vi "Machos.vi"() -> ()   [LabVIEW 2013]
doc: "This example performs a serial port write and a serial port read. The parameters set for the serial port must match the parameters of the connected instrument or device. The VISA Configure Serial Port VI sets the configuration parameters. The front panel displays the controls used to configure the basic parameters, such as baud rate, data bits, and parity. The VI passes the VISA resource name to other VIs that perform operations on that VISA resource. The VISA Write function sends a command to the serial device and the VISA Read function returns data based on the command. The VISA Close function then closes the reference to the serial device. It is important to close the reference; otherwise, further communication through that port might not be possible."
uses:
  <vilib>/Platform/TimedLoop/XDataNode/timing_clust.ctl
  <vilib>/Platform/TimedLoop/XDataNode/nitl_modes.ctl
  <vilib>/Platform/TimedLoop/XDataNode/wakeup.ctl
  <vilib>/Instr/_visa.llb/VISA Configure Serial Port (Instr).vi
  <vilib>/Utility/file.llb/Read From Spreadsheet File (string).vi
  <vilib>/platform/TimedLoop/XDataNode/XDataNode.xnode
  <vilib>/Platform/TimedLoop/XDataNode/XDNodeRunTimeDep.lvlib
panel:
  out "Total":string[](array[string])
  in  "Abrir arnés":bool
  out "Etiquetas":string[](array[string])
  out "Entradas":u8[](array[numeric])
  out "Total":bool[](array[boolean])
  out "Test?":bool[](array[boolean])
  in  "OUTPUT Pin":u8=1 min=1 max=32 step=1
  in  "Puerto":refnum<visa-resource-name>
  out "OK?":bool
  in  "stop":bool
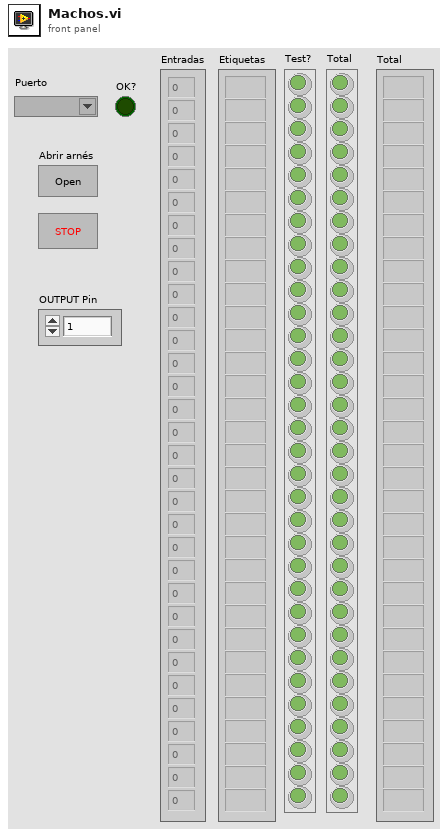
[diagram p1: front panel]
types:
  T1 = typedef "XDNodeRunTimeDep.lvlib/timing_clust.ctl" = cluster{"Expected End [f-1]":u64, "Actual End [f-1]":u64, "Finished Late? [f-1]":bool, "Expected End [i-1]":u64, "Actual End [i-1]":u64, "Finished Late? [i-1]":bool, "Expected Start [i]":u64, "Actual Start [i]":u64, "Expected Start [f]":u64, "Actual Start [f]":u64, "Source Name":string, "Structure Name":string, "Period":i64, "Deadline":i64, "Offset":i64, "Start":i64, "Priority":i32, "Timeout":i32, "Mode":T2, "Wakeup Reason":T3, "Error":errorcluster, "Source Type":string, "Secondary Source Type":string, "Global End Time":u64, "Global Start Time":u64, "Frame Duration":u64, "Iteration Duration":u64, "Assigned CPU":i32, "I/O Scan Engine Mode":u32}
  T2 = typedef "XDNodeRunTimeDep.lvlib/nitl_modes.ctl" = enum32{"No Change", "Process missed periods, maintain original phase", "Discard missed periods, maintain original phase", "Process missed periods, ignore original phase", "Discard missed periods, ignore original phase"}
  T3 = typedef "XDNodeRunTimeDep.lvlib/wakeup.ctl" = enum32{"Normal", "Aborted", "Asynchronous wakeup", "Timing source error", "Timed loop error", "Timeout"}
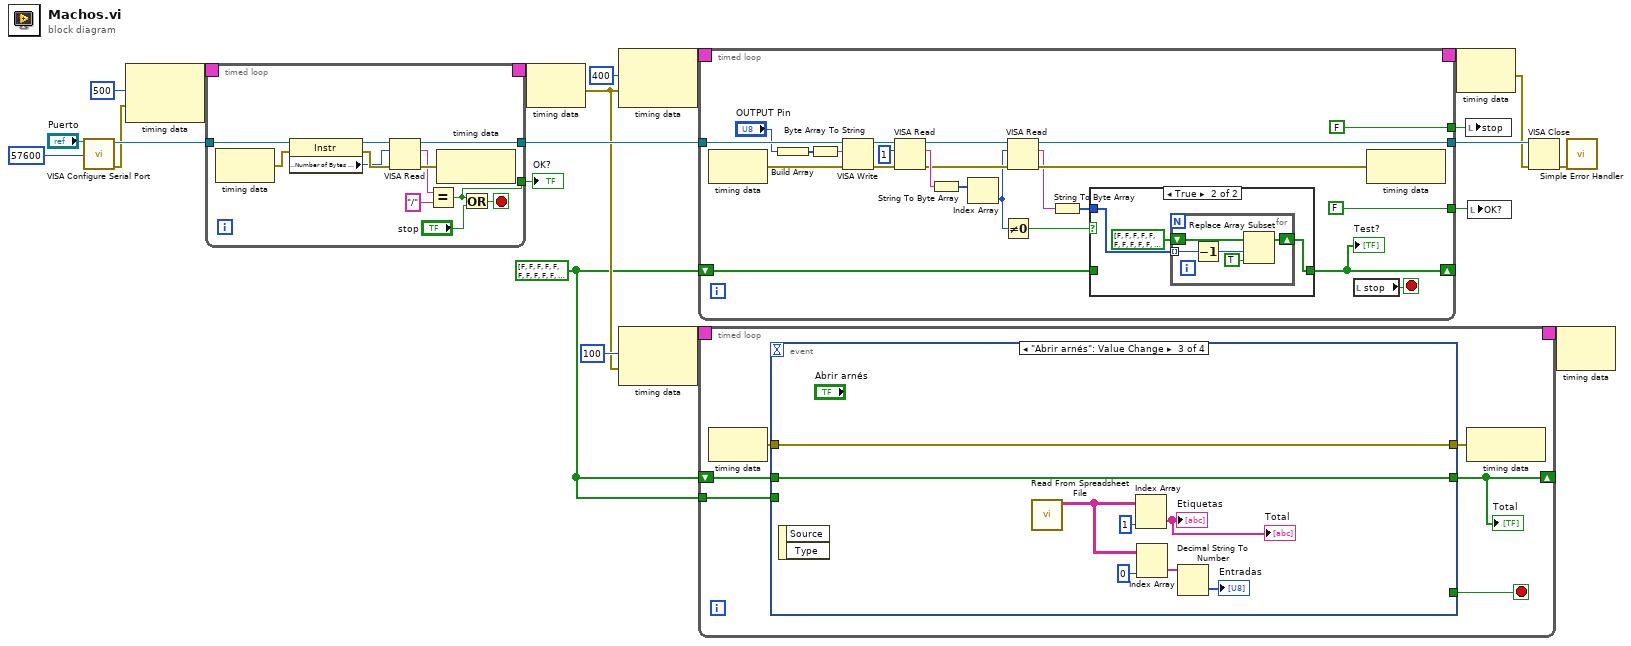
[diagram p0: block diagram]
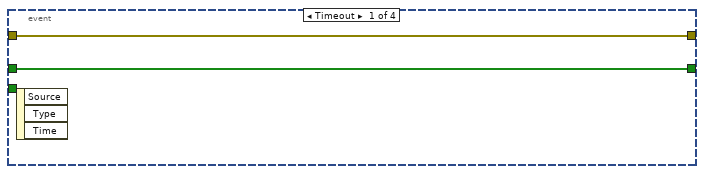
[diagram p2: hidden frame]
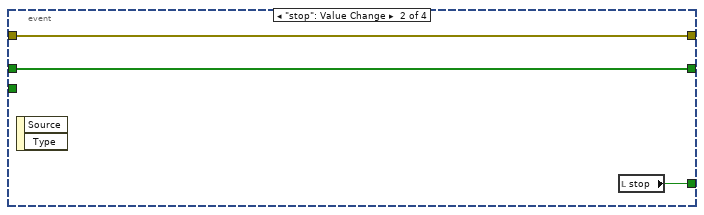
[diagram p3: hidden frame]
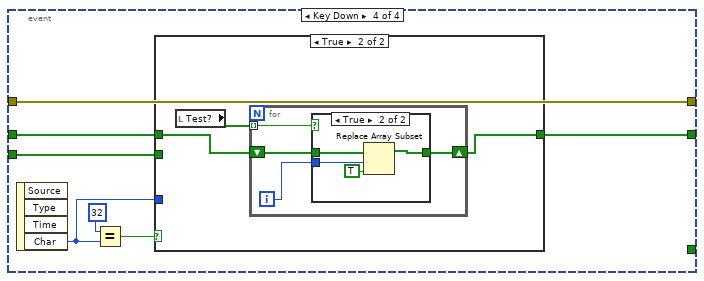
[diagram p4: hidden frame]
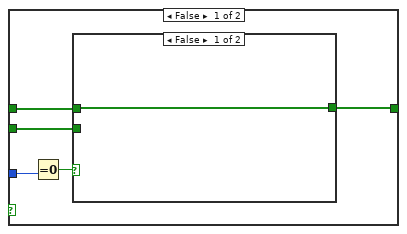
[diagram p5: hidden frame]
diagram:
  w1 = bool[] [FALSE, FALSE, FALSE, FALSE, FALSE, FALSE, FALSE, FALSE, FALSE, FALSE, FALSE, FALSE, FALSE, FALSE, FALSE, FALSE, FALSE, FALSE, FALSE, FALSE, FALSE, FALSE, FALSE, FALSE, FALSE, FALSE, FALSE, FALSE, FALSE, FALSE, FALSE, FALSE, FALSE]
  n1 = call-poly "VISA Configure Serial Port"("VISA resource name"="Puerto", "baud rate (9600)"=u32 57600) -> ("VISA resource name out"=w22:refnum<visa-resource-name>, "error out"=w19:errorcluster)  [unwired: 7 in, 5 out]
  n2 = node-c288(i64 500 ("Period"), w19) -> (w21:T1)
  n3 = timed-loop {
    timing: w21 -> [_]
    timing-out: [_] -> w20
    tunnel: [w34] -> w9
    tunnel: w22 -> [w33]
    tunnel: [w23] -> w12
    stop <- w24 stop-if-true
    n4 = node-c288() -> (w29:errorcluster)  [unwired: 1 in]
    n5 = property class="Instr"(reference=w33, error in=w29) -> (reference out=w32:refnum<visa-resource-name>, error out=w31:errorcluster, "Serial Settings:Number of Bytes at Serial Port"=w30:u32)
    n6 = VISA Read(VISA resource name=w32, byte count=w30, error in (no error)=w31) -> (VISA resource name out=w34:refnum<visa-resource-name>, read buffer=w27:string, error out=w28:errorcluster)  [unwired: 1 out]
    n7 = Equal?(x=w27, y="/") -> (x = y?=w23:bool)
    n8 = node-c288(w28) -> ()  [unwired: 1 out]
    n9 = Or(x=w23, y="stop") -> (x .or. y?=w24:bool)
  }
  "OK?" <- w12
  n10 = node-c288(w20) -> (w2:errorcluster)
  n11 = node-c288(i64 400 ("Period"), w2) -> (w15:T1)
  n12 = node-c288(i64 100 ("Period"), w2) -> (w5:T1)
  n13 = timed-loop {
    timing: w15 -> [_]
    timing-out: [_] -> w14
    tunnel: w9 -> [w62]
    tunnel: [FALSE ("stop")] -> w16
    tunnel: [w60] -> w8
    tunnel: [FALSE ("OK?")] -> w11
    shift-right: [w40] -> _
    shift-left: w1 -> [w43]
    stop <- w41 stop-if-true
    n14 = node-c288() -> (w59:errorcluster)  [unwired: 1 in]
    n15 = Build Array("OUTPUT Pin") -> (w47:u8[])
    n16 = Byte Array To String ("Byte Array \nTo String")(unsigned byte array=w47) -> (string=w46:string)
    n17 = VISA Write(VISA resource name=w62, write buffer=w46, error in (no error)=w59) -> (VISA resource name out=w54:refnum<visa-resource-name>, error out=w53:errorcluster)  [unwired: 1 out]
    n18 = VISA Read(VISA resource name=w54, byte count=u32 1, error in (no error)=w53) -> (VISA resource name out=w49:refnum<visa-resource-name>, read buffer=w55:string, error out=w50:errorcluster)  [unwired: 1 out]
    n19 = String To Byte Array(string=w55) -> (unsigned byte array=w51:u8[])
    n20 = Index Array(array=w51) -> (element=w45:u8)  [unwired: 1 in]
    n21 = Not Equal To 0?(x=w45) -> (x != 0?=w44:bool)
    n22 = VISA Read(VISA resource name=w49, byte count=w45, error in (no error)=w50) -> (VISA resource name out=w60:refnum<visa-resource-name>, read buffer=w48:string, error out=w58:errorcluster)  [unwired: 1 out]
    n23 = String To Byte Array(string=w48) -> (unsigned byte array=w42:u8[])
    n24 = case shown="True" w44 {
      tunnel: w43 -> [w63 _]
      tunnel: [w63 w64] -> w40
      tunnel: w42 -> [_ w66]
      frame False {
      }
      frame True {
        n25 = for {
          tunnel: w66 -> [w68] mode=indexing
          shift-right: [w69] -> w64
          shift-left: bool[] [FALSE, FALSE, FALSE, FALSE, FALSE, FALSE, FALSE, FALSE, FALSE, FALSE, FALSE, FALSE, FALSE, FALSE, FALSE, FALSE, FALSE, FALSE, FALSE, FALSE, FALSE, FALSE, FALSE, FALSE, FALSE, FALSE, FALSE, FALSE, FALSE, FALSE, FALSE, FALSE, FALSE] -> [w70]
          n26 = Decrement(x=w68) -> (x-1=w67:u8)
          n27 = Replace Array Subset(array=w70, new element=TRUE ("new element/subarray"), index=w67) -> (w69:bool[])
        }
      }
    }
    "Test?" <- w40
    n28 = local read "stop"() -> (w41:bool)
    n29 = node-c288(w58) -> ()  [unwired: 1 out]
  }
  n30 = timed-loop {
    timing: w5 -> [_]
    timing-out: [_] -> w4
    shift-right: [w78] -> _
    shift-left: w1 -> [w79]
    tunnel: w1 -> [w77]
    stop <- w80 stop-if-true
    n31 = node-c288() -> (w82:errorcluster)  [unwired: 1 in]
    n32 = event shown="[2] \"Abrir arnés\": Value Change" {
      selector: _ -> [_ _ _ _]
      dyn-events: _ -> [_ _ _ _]
      timeout: _ -> [_ _ _ _]
      tunnel: w82 -> [w84 w86 w93 w102]
      tunnel: [w84 w86 w93 w102] -> w81
      tunnel: [_ w87 _ _] -> w80
      tunnel: w79 -> [w83 w85 w89 w101]
      tunnel: [w83 w85 w89 w100] -> w78
      tunnel: w77 -> [_ _ _ w97]
      event Timeout {
        n33 = event-data() -> ()  [unwired: 1 in, 3 out]
      }
      event "stop": Value Change {
        n34 = event-data() -> ()  [unwired: 1 in, 2 out]
        n35 = local read "stop"() -> (w87:bool)
      }
      event "Abrir arnés": Value Change {
        n36 = event-data() -> ()  [unwired: 1 in, 2 out]
        n37 = call-poly <vilib>:"Read From Spreadsheet File.vi"() -> ("all rows"=w95:string[][])  [unwired: 7 in, 4 out]
        n38 = Index Array(array=w95, index (col)=1 ("index (row)")) -> (element=→"Etiquetas" →"Total":string[])  [unwired: 1 in]
        n39 = Index Array(array=w95, index (col)=0 ("index (row)")) -> (element=w92:string[])  [unwired: 1 in]
        n40 = Decimal String To Number(string=w92) -> (number=→"Entradas":i32[])  [unwired: 2 in, 1 out]
      }
      event Key Down {
        n41 = event-data() -> ("Char"=w96:i16)  [unwired: 1 in, 3 out]
        n42 = Equal?(x=i16 32, y=w96) -> (x = y?=w98:bool)
        n43 = case shown="True" w98 {
          tunnel: w101 -> [w104 w111]
          tunnel: [w103 w110] -> w100
          tunnel: w97 -> [w105 _]
          tunnel: w96 -> [w107 _]
          frame False {
            n44 = Equal To 0?(x=w107) -> (x = 0?=w106:bool)
            n45 = case shown="False" w106 {
              tunnel: w105 -> [_ w109]
              tunnel: [w108 w109] -> w103
              tunnel: w104 -> [w108 _]
              frame False {
              }
              frame True {
              }
            }
          }
          frame True {
            n46 = local read "Test?"() -> (w112:bool[])
            n47 = for {
              tunnel: w112 -> [w116] mode=indexing
              shift-right: [w114] -> w110
              shift-left: w111 -> [w115]
              i -> [w113]
              n48 = case shown="True" w116 {
                tunnel: w115 -> [w117 w120]
                tunnel: [w117 w119] -> w114
                tunnel: w113 -> [_ w118]
                frame False {
                }
                frame True {
                  n49 = Replace Array Subset(array=w120, new element=TRUE ("new element/subarray"), index=w118) -> (w119:bool[])
                }
              }
            }
          }
        }
      }
    }
    "Total" <- w78
    n50 = node-c288(w81) -> ()  [unwired: 1 out]
  }
  n51 = node-c288(w14) -> (w7:errorcluster)
  n52 = local write "stop"(w16) -> ()
  n53 = local write "OK?"(w11) -> ()
  n54 = VISA Close(VISA resource name=w8, error in (no error)=w7) -> (error out=w17:errorcluster)
  n55 = node-c288(w4) -> ()  [unwired: 1 out]
  n56 = call <vilib>:"Simple Error Handler.vi"("error in (no error)"=w17) -> ()  [unwired: 4 in, 5 out]
